vi "CleanUp.vi"(8 "Error In":errorcluster, 11 "Object in":refnum<class "Scope.lvclass">) -> (0 "Error Out":errorcluster, 3 "object out":refnum<class "Scope.lvclass">)   [LabVIEW 2023, in "HAL.lvlib" / "Scope.lvclass"]
uses:
  Scope.lvclass
  Hardware_class/Hardware.lvclass
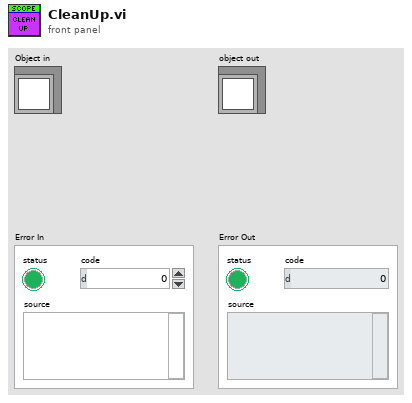
[diagram p1: front panel]
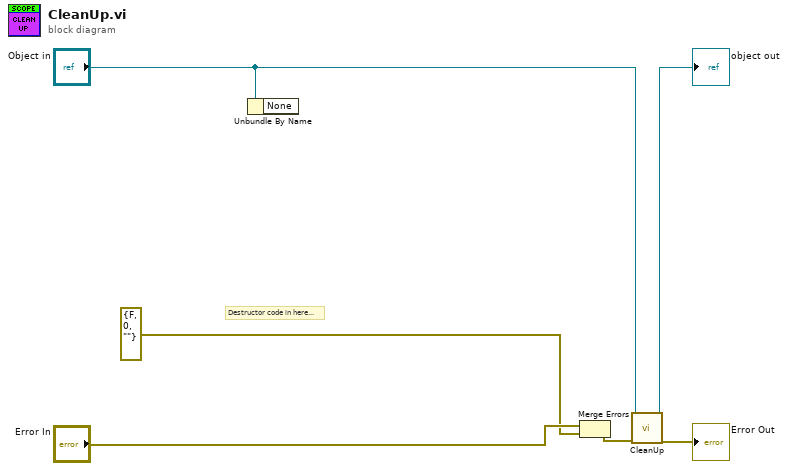
[diagram p0: block diagram]
diagram:
  # "Destructor code in here..."
  n1 = Unbundle By Name("Object in") -> ()  [unwired: 1 out]
  n2 = Merge Errors("Error In", errorcluster {"status"=FALSE, "code"=0, "source"=""} ("error in (no error)")) -> (w2:errorcluster)
  n3 = call-parent "CleanUp.vi"("Error In"=w2, "object in"="Object in") -> ("Error Out"=→"Error Out":errorcluster, "object out"=→"object out":refnum<class "Scope.lvclass">)  [unwired: 8 in]
